vi "Enum Conversion Paths.vi"(8 "error in (no error)":errorcluster, 10 "Enum Type Name":string, 11 "LV-Protoc in":refnum<class "LV-Protoc.lvclass">) -> (0 "error out":errorcluster, 1 "Enum from Value Path":path, 2 "Enum Value Path":path, 3 "LV-Protoc out":refnum<class "LV-Protoc.lvclass">)   [LabVIEW 2020, in "LV-Protoc.lvlib" / "LV-Protoc.lvclass"]
uses:
  LV-Protoc.lvclass
  LV-Protoc.lvclass/LV-Protoc.ctl
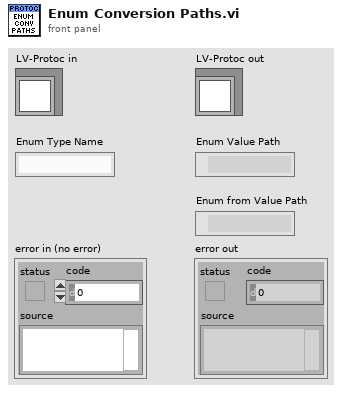
[diagram p1: front panel]
types:
  T1 = typedef "LV-Protoc.lvlib/Enumeration Paths.ctl" = cluster{"Name":string, "Typedef Path":path, "Enum to Value Path":path, "Enum from Value Path":path, "Library Path":path}
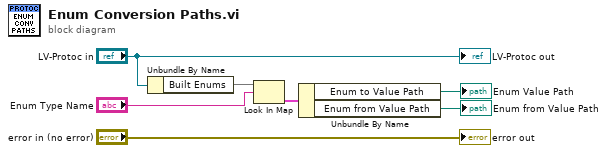
[diagram p0: block diagram]
diagram:
  n1 = Unbundle By Name("LV-Protoc in") -> ("Built Enums"=w7:map{string, T1})
  n2 = Look In Map(map=w7, key="Enum Type Name") -> (value=w6:T1)  [unwired: 1 in, 1 out]
  n3 = Unbundle By Name(w6) -> ("Enum to Value Path"=→"Enum Value Path":path, "Enum from Value Path"=→"Enum from Value Path":path)
  "error out" <- "error in (no error)"
  "LV-Protoc out" <- "LV-Protoc in"
